vi "B_WriteClassAttribute.vi"(0 "reference in":refnum<class "BaseTemplate.lvclass">, 5 "error in (no error)":errorcluster) -> (14 "reference out":refnum<class "BaseTemplate.lvclass">, 19 "error out":errorcluster)   [LabVIEW 2016, in "BaseTemplate.lvclass"]
uses:
  <resource>/Framework/Providers/Open_GDS/ClassProviders/Provider_EndevoGOOP300/Templates/BaseTemplate/BaseTemplate.lvclass
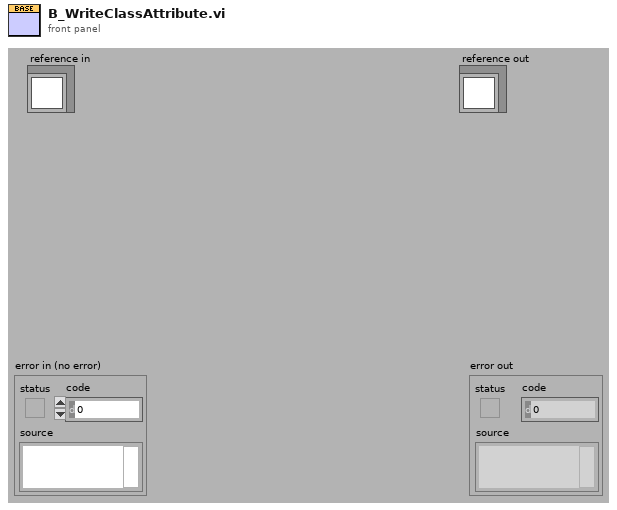
[diagram p1: front panel]
types:
  T1 = typedef "BaseTemplate.lvclass/ClassAttributes.ctl" = cluster{"classAttribute1":bool}
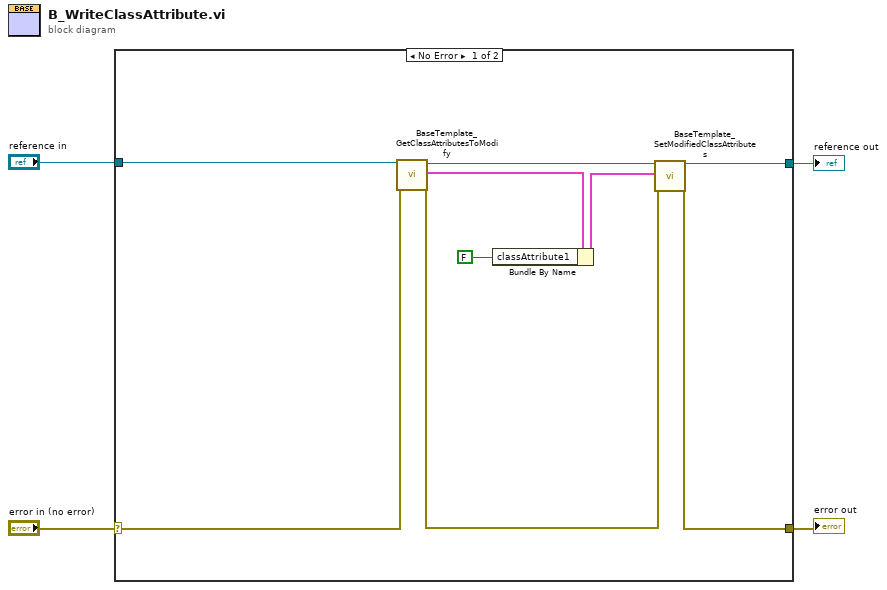
[diagram p0: block diagram]
diagram:
  n1 = case shown="No Error" "error in (no error)" {
    selector: "error in (no error)" -> [w6 w15]
    tunnel: [w10 w15] -> w3
    tunnel: [w9 w14] -> w1
    tunnel: "reference in" -> [w5 w14]
    frame No Error {
      n2 = call <resource>:"BaseTemplate_GetClassAttributesToModify.vi"("reference in"=w5, "error in (no error)"=w6) -> ("reference out"=w11:refnum<class "BaseTemplate.lvclass">, "Class attributes"=w13:T1, "error out"=w8:errorcluster)  [unwired: 14 in, 1 out]
      n3 = Bundle By Name(cluster=w13, "classAttribute1"=FALSE) -> (w12:T1)
      n4 = call <resource>:"BaseTemplate_SetModifiedClassAttributes.vi"("reference in"=w11, "Class attributes"=w12, "error in (no error)"=w8) -> ("reference out"=w9:refnum<class "BaseTemplate.lvclass">, "error out"=w10:errorcluster)  [unwired: 15 in]
    }
    frame Error {
    }
  }
  "error out" <- w3
  "reference out" <- w1
